vi "Configure Frequency Modulation.vi"(7 "Frequency (0.1 Hz)":dbl=0.1, 8 "error in (no error)":errorcluster, 9 "Deviation (0 Hertz)":dbl, 10 "Enable Frequency Modulation (0: Off)":bool, 11 "VISA resource name":refnum<visa-resource-name>) -> (0 "error out":errorcluster, 3 "VISA resource name out":refnum<visa-resource-name>)   [LabVIEW 2020, in "Agilent 681x Series.lvlib"]
doc: "Configures the frequency modulation of output frequency. \n\nNote: \nFrequency modulation operates only, If <b>FREQuency:MODE</b> is set to Fixed mode in <b>Configure Output Frequency.vi</b>."
uses:
  <instrlib>/Agilent 681x Series/Agilent 681x Series.lvlib
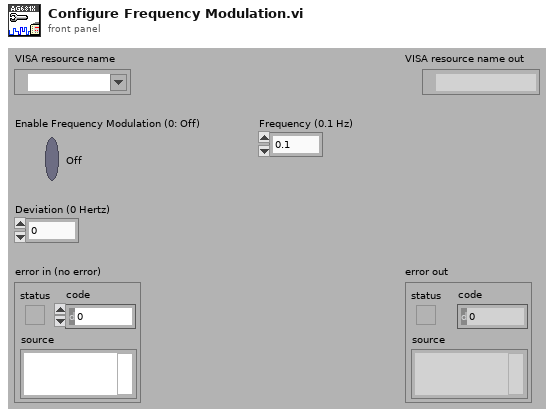
[diagram p1: front panel]
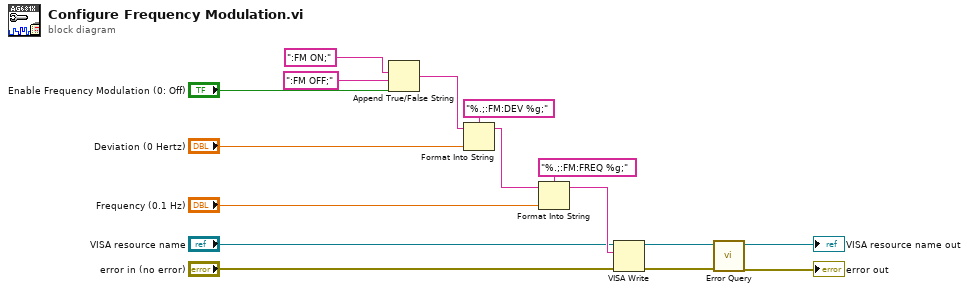
[diagram p0: block diagram]
diagram:
  n1 = Append True/False String(1:"Enable Frequency Modulation (0: Off)", 2:":FM OFF;", 3:":FM ON;") -> (0:w14:string)  [unwired: 1 in]
  n2 = Format Into String(format string="%.;:FM:DEV %g;", initial string=w14, "Deviation (0 Hertz)") -> (resulting string=w11:string)  [unwired: 1 in, 1 out]
  n3 = Format Into String(format string="%.;:FM:FREQ %g;", initial string=w11, "Frequency (0.1 Hz)") -> (resulting string=w8:string)  [unwired: 1 in, 1 out]
  n4 = VISA Write(VISA resource name="VISA resource name", write buffer=w8, error in (no error)="error in (no error)") -> (VISA resource name out=w5:refnum<visa-resource-name>, error out=w4:errorcluster)  [unwired: 1 out]
  n5 = call <instrlib>:"Error Query.vi"("error in (no error)"=w4, "VISA resource name"=w5) -> ("error out"=→"error out":errorcluster, "VISA resource name out"=→"VISA resource name out":refnum<visa-resource-name>)  [unwired: 6 in, 2 out]
